vi "DecodeUInt32.vi"(1 "Data In":u8[](array[numeric])) -> (0 "Data Out":u32[](array[numeric]))   [LabVIEW 2015, in "navX Library v1 (deprecated).lvlib"]
uses:
  navX Library v1 (deprecated).lvlib
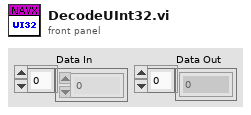
[diagram p1: front panel]
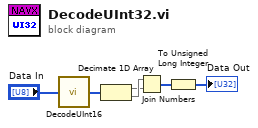
[diagram p0: block diagram]
diagram:
  n1 = call "DecodeUInt16.vi"("Data In"="Data In") -> ("Data Out"=w5:u16[])
  n2 = Decimate 1D Array(w5) -> (w3:u16[], w4:u16[])
  n3 = Join Numbers(hi=w4, lo=w3) -> ((hi.lo)=w2:u32[])
  n4 = To Unsigned Long Integer(number=w2) -> (unsigned 32bit integer=→"Data Out":u32[])
